vi "Write Actors.vi"(8 "error in (no error)":errorcluster, 10 "Actors":refnum<class "CS++Actor.lvclass">[](array[class]), 11 "CS++MessageMakerMain in":refnum<class "CS++MessageMakerMain.lvclass">) -> (0 "error out":errorcluster, 3 "CS++MessageMakerMain out":refnum<class "CS++MessageMakerMain.lvclass">)   [LabVIEW 2014, in "CS++MessageMakerMain.lvlib" / "CS++MessageMakerMain.lvclass"]
uses:
  CS++MessageMakerMain.lvclass
  CSPP_Actor/CS++Actor.lvclass
  CS++MessageMakerMain.lvclass/CS++MessageMakerMain.ctl
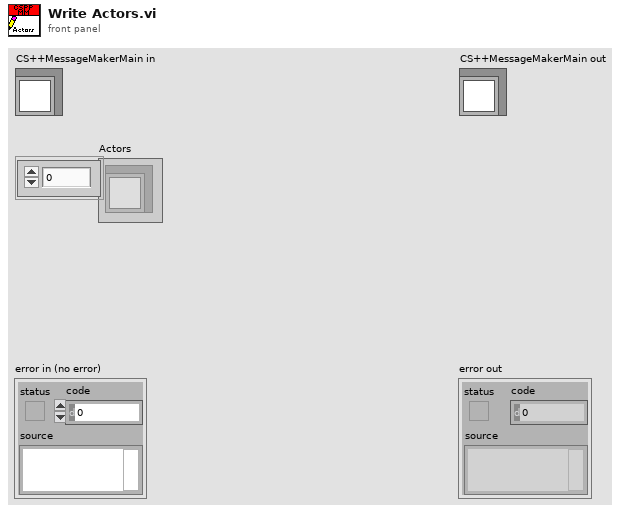
[diagram p1: front panel]
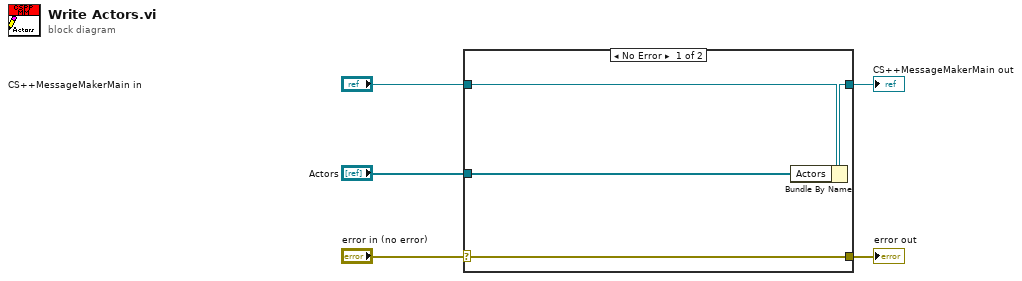
[diagram p0: block diagram]
diagram:
  n1 = case shown="No Error" "error in (no error)" {
    selector: "error in (no error)" -> [w9 w10]
    tunnel: [w9 w10] -> w4
    tunnel: [w7 w11] -> w2
    tunnel: "CS++MessageMakerMain in" -> [w8 w11]
    tunnel: "Actors" -> [w6 _]
    frame No Error {
      n2 = Bundle By Name(cluster=w8, "Actors"=w6) -> (w7:refnum<class "CS++MessageMakerMain.lvclass">)
    }
    frame Error {
    }
  }
  "error out" <- w4
  "CS++MessageMakerMain out" <- w2
